vi "Data Conversion for Read Data.vi"(10 "data out":string, 11 "Read Data Type":enum16{"String", "Intiger", "DBL", "SGL"}(ring)) -> (1 "Data regiter":sgl[](array[numeric]), 2 "M Intiger":u16[](array[numeric]), 3 "String":string, 5 "String Array":string[](array[string]))   [LabVIEW 2024]
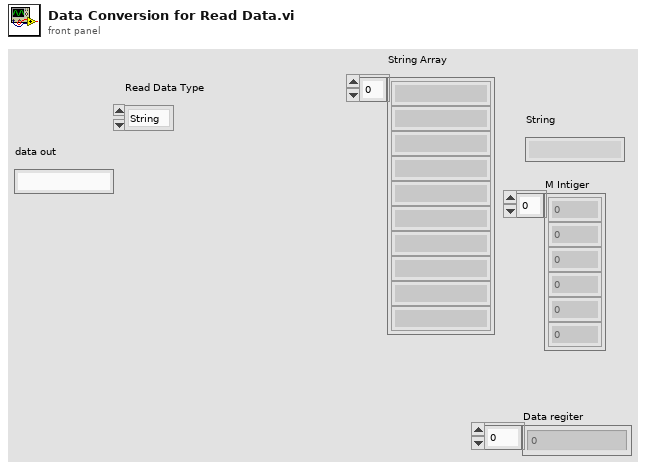
[diagram p1: front panel]
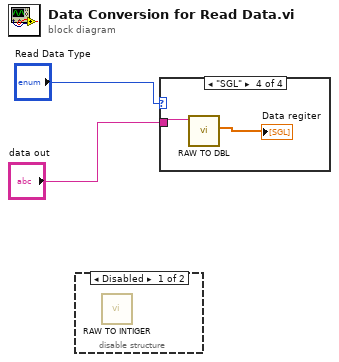
[diagram p0: block diagram]
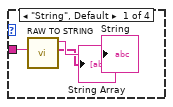
[diagram p3: hidden frame]
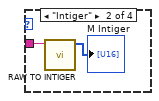
[diagram p4: hidden frame]
diagram:
  n1 = disable-structure shown="Disabled" {
    frame Disabled {
      n2 = call "RAW TO INTIGER.vi"() -> ()  [unwired: 10 in, 2 out]
    }
    frame Enabled {
    }
  }
  n3 = case shown="\"SGL\"" "Read Data Type" {
    tunnel: "data out" -> [w5 w6 _ w9]
    frame "String", Default {
      n4 = call "RAW TO STRING.vi"("data out"=w5) -> ("String Array"=→"String Array":string[], "String"=→"String":string)  [unwired: 9 in]
    }
    frame "Intiger" {
      n5 = call "RAW TO INTIGER.vi"("data in"=w6) -> ("INITEER"=→"M Intiger":u16[])  [unwired: 9 in, 1 out]
    }
    frame "DBL" {
    }
    frame "SGL" {
      n6 = call "RAW TO DBL.vi"("data in"=w9) -> ("Data regiter (SGL)"=→"Data regiter":sgl[])  [unwired: 8 in, 2 out]
    }
  }
